vi "test图层-修改中.vi"() -> ()   [LabVIEW 2018]
doc: "This example demonstrates the use of binary morphological reconstruction in the particle analysis. The example allows you to keep the particles completely inside the ROI, completely outside the ROI or on the ROI."
uses:
  <vilib>/vision/NI_Vision_Development_Module.lvlib
panel:
  out "Image Compare":T1(plugin-control)
  out "下":i32
  out "右":i32
  out "上":i32
  out "左":i32
  out "面积":i32
  out "标准差":sgl
  out "平均值":sgl
  out "最大灰度值":sgl
  out "最小灰度值":sgl
  out "选中框灰度表":u32[](graph)
  out "Image Dst Out":T1(plugin-control)
  out "全图灰度级信息":T2 {"标准差" format="%.2f"; "均值" format="%.2f"; "相邻灰度级间隔" format="%.2f"; "起始灰度值" format="%.2f"; "最大值" format="%.2f"; "最小值" format="%.2f"}
  out "图片灰度表":u32[](graph)
  in  "Font, Size & Style 2":T3={"Desired Font (Application)"=enum."Application Font", "[User-specified Font]"={"Font Name"="", "Size"=12, "Strikeout?"=FALSE, "Italic?"=FALSE, "Underline?"=FALSE, "Outline?"=FALSE, "Shadow?"=FALSE, "Bold?"=FALSE, "Rotation Angle"=0.0}, "Horizontal Alignment"=0, "Vertical Alignment"=0} {"Vertical Alignment" items=["Bottom", "Top", "Baseline"]; "Horizontal Alignment" items=["Left", "Center", "Right"]; "[User-specified Font]"."Rotation Angle" format="%.2f"}
  in  "选择框号":bool
  out "当前选择框的编号":dbl
  out "框总数":dbl
  in  "Font, Size & Style":T3={"Desired Font (Application)"=enum."Application Font", "[User-specified Font]"={"Font Name"="", "Size"=12, "Strikeout?"=FALSE, "Italic?"=FALSE, "Underline?"=FALSE, "Outline?"=FALSE, "Shadow?"=FALSE, "Bold?"=FALSE, "Rotation Angle"=0.0}, "Horizontal Alignment"=0, "Vertical Alignment"=0} {"Vertical Alignment" items=["Bottom", "Top", "Baseline"]; "Horizontal Alignment" items=["Left", "Center", "Right"]; "[User-specified Font]"."Rotation Angle" format="%.2f"}
  out "框组":T4(array[cluster])
  in  "单次删除":bool
  in  "Operation":enum16{"overlay rectangle"}(ring)
  out "标注图":T1(plugin-control)
  in  "退出标注":bool
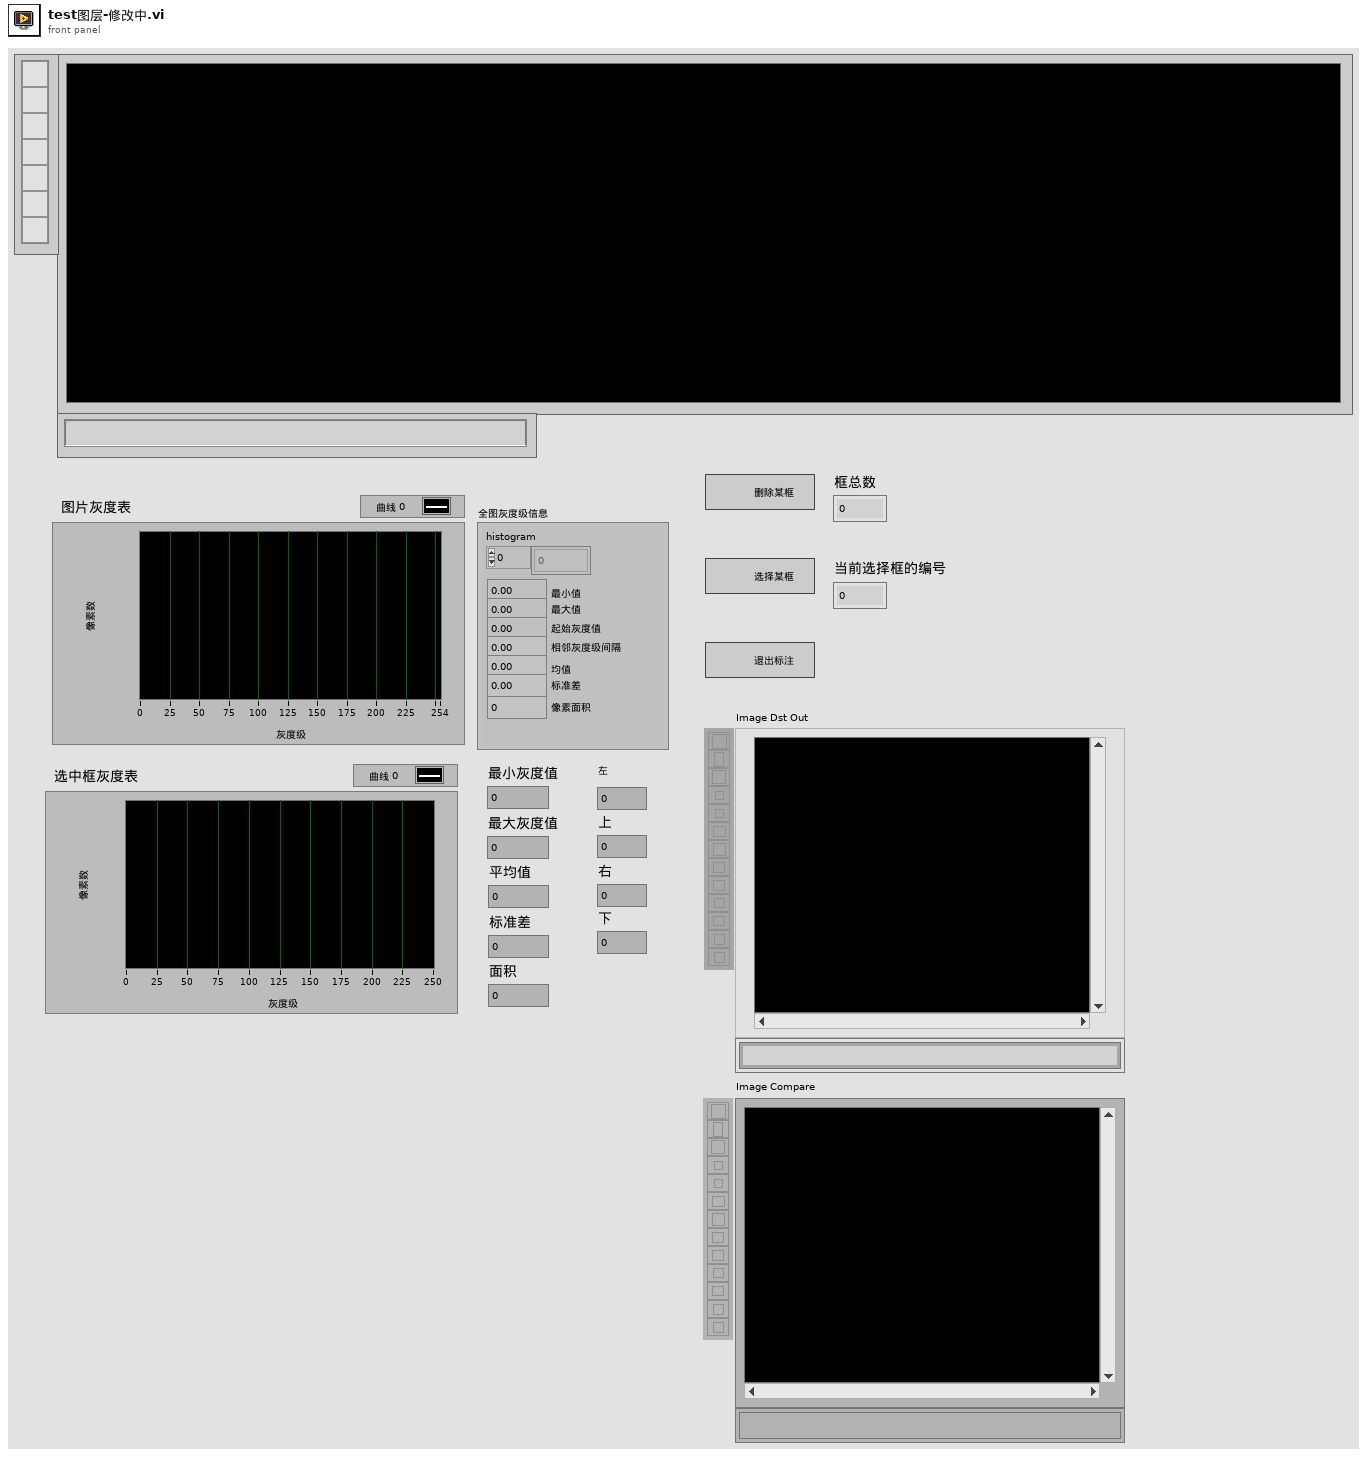
[diagram p1: front panel]
types:
  T1 = typedef "IMAQ Image.ctl" = refnum<image>
  T2 = cluster{"histogram":u32[], "最小值":sgl, "最大值":sgl, "起始灰度值":sgl, "相邻灰度级间隔":sgl, "均值":sgl, "标准差":sgl, "像素面积":i32}
  T3 = cluster{"Desired Font (Application)":enum16{"User-specified Font", "Application Font", "System Font", "Dialog Font"}, "[User-specified Font]":cluster{"Font Name":string, "Size":i16, "Strikeout?":bool, "Italic?":bool, "Underline?":bool, "Outline?":bool, "Shadow?":bool, "Bold?":bool, "Rotation Angle":dbl}, "Horizontal Alignment":i16, "Vertical Alignment":i16}
  T4 = cluster{"Global Rectangle":i32[], "Contours":cluster{"Contour Type":u32, "ROI Type":u32, "Points":i32[]}[]}[]
  T5 = typedef "Image Type" = u32
  T6 = enum32{"Average", "Min", "Max", "Clear  if < ", "Clear  if < or =", "Clear  if =", "Clear  if > or =", "Clear  if >"}
  T7 = cluster{"Global Rectangle":i32[], "Contours":cluster{"Contour Type":u32, "ROI Type":u32, "Points":i32[]}[]}
  T8 = typedef "IMAQ Rectangle" = cluster{"Left":i32, "Top":i32, "Right":i32, "Bottom":i32, "Rotation":dbl}
  T9 = cluster{"histogram":u32[], "Minimal Value":sgl, "Maximal Value":sgl, "Starting Value":sgl, "Interval Width":sgl, "Mean Value":sgl, "Standard  Variation":sgl, "Area (pixels)":i32}
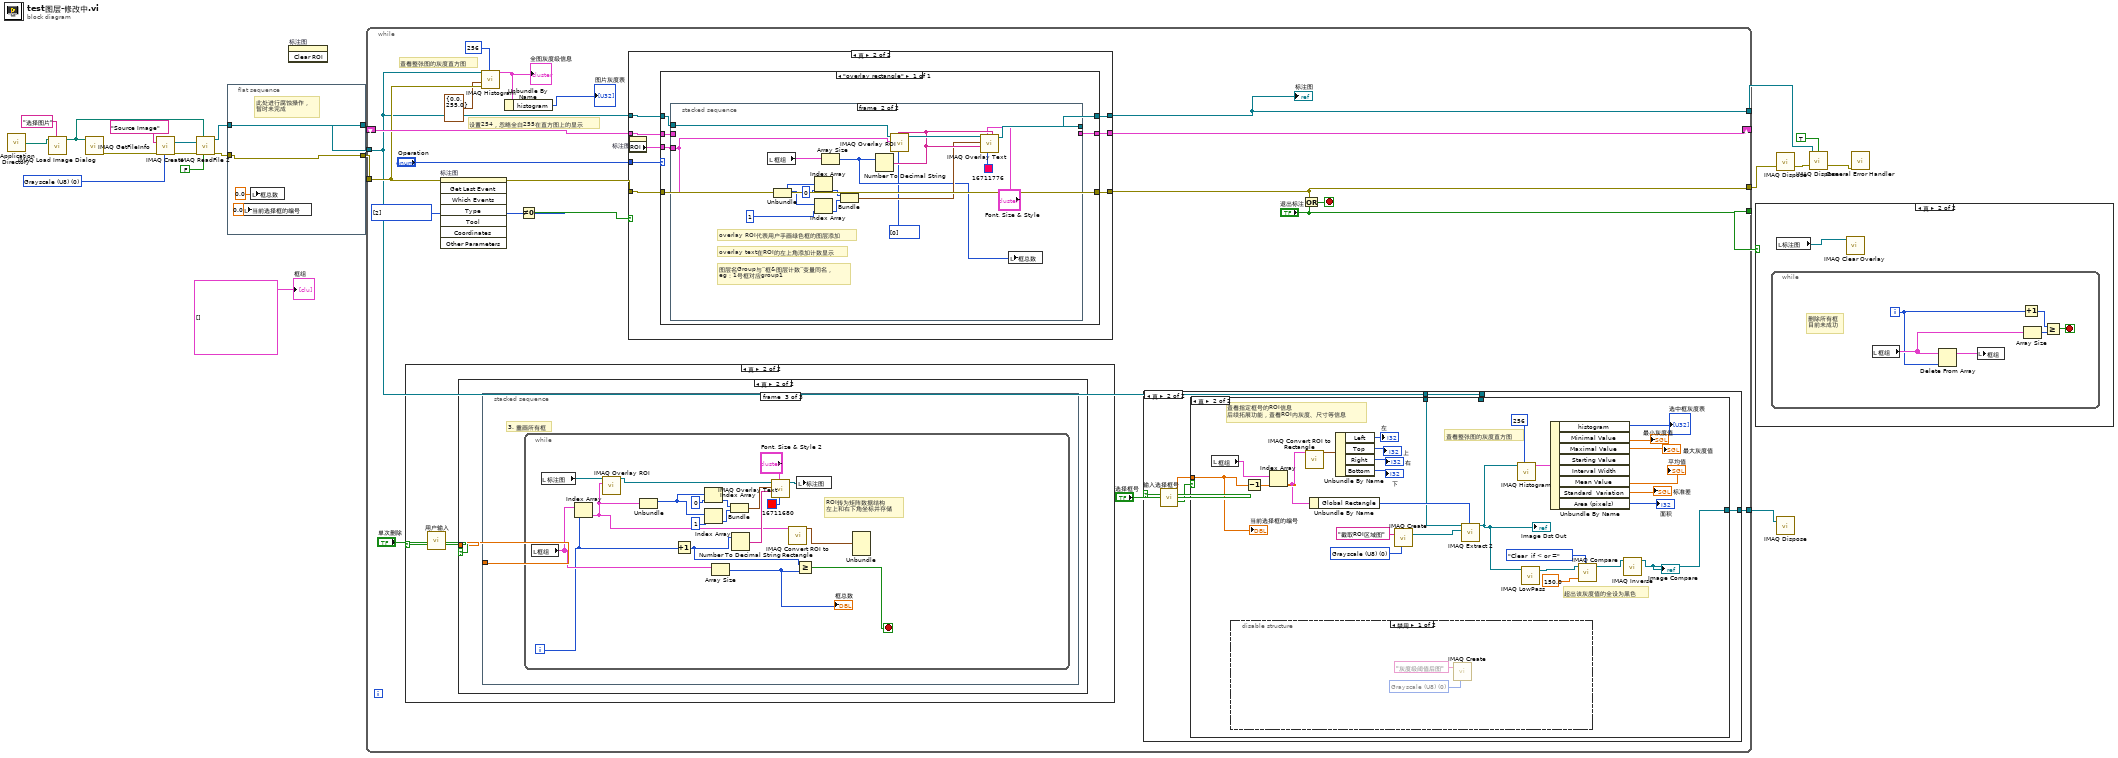
[diagram p0: block diagram]
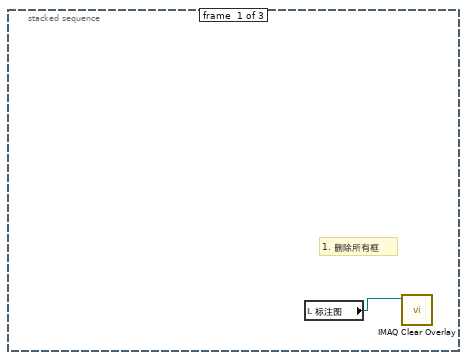
[diagram p8: hidden frame]
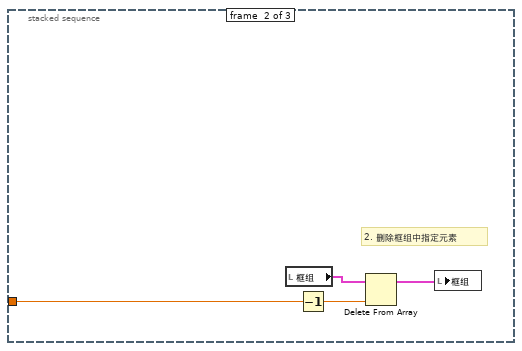
[diagram p9: hidden frame]
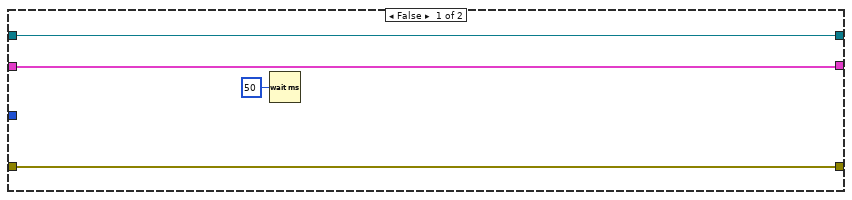
[diagram p10: hidden frame]
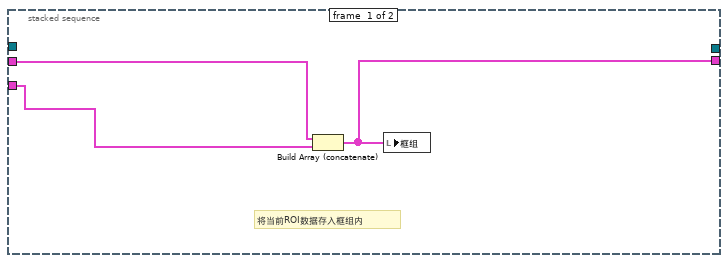
[diagram p11: hidden frame]
diagram:
  w12 = T5 0 items=["Grayscale (U8)", "Grayscale (I16)", "Grayscale (SGL)", "Complex (CSG)", "RGB (U32)", "HSL (U32)", "RGB (U64)", "Grayscale (U16)"] ("Image Type")
  n1 = call <vilib>:"Application Directory.vi"() -> ("Application Directory"=w13:path)
  n2 = call "IMAQ Load Image Dialog"("Prompt"="选择图片" ("prompt"), "Start Path"=w13) -> ("Path"=w19:path)  [unwired: 7 in, 2 out]
  n3 = call "IMAQ GetFileInfo"("File Path"=w19) -> ("error out"=w17:errorcluster)  [unwired: 4 in, 6 out]
  n4 = call "IMAQ Create"("Image Name"="Source Image", "Image Type"=w12, "error in (no error)"=w17) -> ("New Image"=w15:T1, "error out"=w14:errorcluster)  [unwired: 2 in]
  n5 = call "IMAQ ReadFile 2"("Use File Path Image Type"=FALSE, "File Path"=w19, "error in (no error)"=w14, "Image"=w15) -> ("error out"=w4:errorcluster, "Image Out"=w2:T1)  [unwired: 3 in, 3 out]
  n6 = flat-sequence {
    tunnel: [w23] -> w3
    tunnel: w4 -> [w23]
    tunnel: w2 -> [w22]
    tunnel: [w22] -> w1
    frame #0 {
      # "此处进行腐蚀操作，\n暂时未完成"
      n7 = local write "当前选择框的编号"(0.0 ("当前框的编号")) -> ()
      n8 = local write "框总数"(0.0 ("框总数")) -> ()
    }
  }
  n9 = invoke on="标注图" class="ImageControl" method="Clear ROI"() -> ()  [unwired: 3 in, 3 out]
  n10 = while {
    tunnel: [w28] -> w10
    tunnel: [w41] -> w8
    shift-right: [w37] -> _
    shift-left: _ -> [w36]
    tunnel: ["退出标注"] -> w20
    tunnel: w3 -> [w33]
    tunnel: [w27] -> w5
    tunnel: w1 -> [w26]
    stop <- w40 stop-if-true
    w43 = i32[] [2] items=["No Event"=0, "Click Event"=1, "Draw Event"=2, "Size Event"=4, "Scroll Event"=5, "Double Click Event"=8] ("Which Events")
    # "设置254，忽略全白255在直方图上的显示"
    # "查看整张图的灰度直方图"
    n11 = case shown="真" "单次删除" {
      frame False {
      }
      frame True {
        n12 = call "用户输入"() -> ("框号"=w83:dbl, "确定"=w84:bool)  [unwired: 17 in, 1 out]
        n13 = case shown="真" w84 {
          tunnel: w83 -> [_ w85]
          frame False {
            # "用户取消操作"
          }
          frame True {
            n14 = stacked-sequence {
              tunnel: w85 -> [_ w89 _]
              frame #0 {
                # "1. 删除所有框"
                n15 = local read "标注图"() -> (w86:T1)
                n16 = call "IMAQ Clear Overlay"("Image"=w86) -> ()  [unwired: 9 in, 2 out]
              }
              frame #1 {
                # "2. 删除框组中指定元素"
                n17 = local read "框组"() -> (w90:T4)
                n18 = Decrement(x=w89) -> (x-1=w88:dbl)
                n19 = Delete From Array(array=w90, index=w88) -> (array with subset deleted=w87:T4)  [unwired: 1 in, 1 out]
                n20 = local write "框组"(w87) -> ()
              }
              frame #2 {
                # "3. 重画所有框"
                n21 = while {
                  i -> [w94]
                  stop <- w109 stop-if-true
                  # "ROI转为矩阵数据结构\n左上和右下角坐标并存储"
                  n22 = local read "框组"() -> (w102:T4)
                  n23 = local read "标注图"() -> (w108:T1)
                  n24 = Index Array(array=w102, index=w94) -> (element=w95:T7)
                  n25 = call "IMAQ Overlay ROI"("ROI Descriptor"=w95, "Image"=w108) -> ("Image Out"=w104:T1)  [unwired: 8 in, 1 out]
                  n26 = Unbundle(w95) -> ("Global Rectangle"=w98:i32[])  [unwired: 1 out]
                  n27 = Increment(x=w94) -> (x+1=w107:i32)
                  n28 = Index Array(array=w98, index=0 ("索引")) -> (element=w99:i32)
                  n29 = Index Array(array=w98, index=1 ("索引")) -> (element=w100:i32)
                  n30 = Array Size(array=w102) -> (size(s)=w92:i32)
                  "框总数" <- w92
                  n31 = Bundle(w99, w100) -> (w97:cluster{i32, i32})  [unwired: 1 in]
                  n32 = Number To Decimal String(number=w107) -> (decimal integer string=w105:string)  [unwired: 1 in]
                  n33 = call "IMAQ Overlay Text"("Text Color (black)"=u32 16711680, "Font, Size & Style"="Font, Size & Style 2", "String"=w105, "Origin"=w97, "Image"=w104) -> ("Image Out"=w103:T1)  [unwired: 5 in, 1 out]
                  n34 = call "IMAQ Convert ROI to Rectangle"("ROI Descriptor"=w95) -> ("Rectangle"=w93:T8)  [unwired: 8 in, 1 out]
                  n35 = Greater Or Equal?(x=w107, y=w92) -> (x >= y?=w109:bool)
                  n36 = local write "标注图"(w103) -> ()
                  n37 = Unbundle(w93) -> ()  [unwired: 5 out]
                }
              }
            }
          }
        }
      }
    }
    n38 = invoke on="标注图" class="ImageControl" method="Get Last Event"(error in=w33, "Which Events"=w43) -> (error out=w42:errorcluster, "Type"=w44:i32)  [unwired: 6 in, 6 out]
    n39 = call "IMAQ Histogram"("Number of Classes"=256, "error in (no error)"=w33, "Interval Range"=cluster{"Minimum":sgl, "Maximum":sgl} {"Minimum"=0.0, "Maximum"=255.0}, "Image"=w26) -> ("Histogram Report"=w30:T9)  [unwired: 6 in, 1 out]
    "全图灰度级信息" <- w30
    n40 = Unbundle By Name(w30) -> ("histogram"=→"图片灰度表":u32[])
    n41 = Not Equal To 0?(x=w44) -> (x != 0?=w38:bool)
    n42 = case shown="真" w38 {
      tunnel: w26 -> [w113 w121]
      tunnel: [w113 w120] -> w28
      tunnel: "Operation" -> [_ w118]
      tunnel: w42 -> [w112 w117]
      tunnel: [w112 w116] -> w41
      tunnel: [w110 w115] -> w37
      tunnel: w36 -> [w110 w114]
      frame False {
        n43 = Wait (ms)(milliseconds to wait=u32 50) -> ()  [unwired: 1 out]
      }
      frame True {
        n44 = property on="标注图" class="ImageControl"() -> ("ROI"=w119:T7)  [unwired: 2 in, 2 out]
        n45 = case shown="\"overlay rectangle\"" w118 {
          tunnel: w121 -> [w126]
          tunnel: w119 -> [w124]
          tunnel: [w125] -> w120
          tunnel: w117 -> [w127]
          tunnel: [w127] -> w116
          tunnel: [w123] -> w115
          tunnel: w114 -> [w122]
          frame "overlay rectangle" {
            n46 = stacked-sequence {
              tunnel: w126 -> [_ w137]
              tunnel: [_ w136] -> w125
              tunnel: w124 -> [w130 w133]
              tunnel: [w128 _] -> w123
              tunnel: w122 -> [w129 _]
              frame #0 {
                # "将当前ROI数据存入框组内"
                n47 = Build Array (concatenate)(w129, w130) -> (w128:T4)
                n48 = local write "框组"(w128) -> ()
              }
              frame #1 {
                # "图层名Group与“框&图层计数”变量同名，\neg：1号框对应group1"
                # "overlay text在ROI的左上角添加计数显示"
                # "overlay ROI代表用户手画绿色框的图层添加"
                n49 = local read "框组"() -> (w142:T4)
                n50 = Unbundle(w133) -> ("Global Rectangle"=w145:i32[])  [unwired: 1 out]
                n51 = Index Array(array=w145, index=0 ("索引")) -> (element=w144:i32)
                n52 = Index Array(array=w145, index=1 ("索引")) -> (element=w143:i32)
                n53 = Array Size(array=w142) -> (size(s)=w132:i32)
                n54 = Bundle(w144, w143) -> (w135:cluster{i32, i32})  [unwired: 1 in]
                n55 = Number To Decimal String(number=w132) -> (decimal integer string=w141:string)  [unwired: 1 in]
                n56 = call "IMAQ Overlay ROI"("Colors (Green)"=u32[] [0], "Group"=w141, "ROI Descriptor"=w133, "Image"=w137) -> ("Image Out"=w146:T1)  [unwired: 6 in, 1 out]
                n57 = call "IMAQ Overlay Text"("Group"=w141, "Text Color (black)"=u32 16711776, "Font, Size & Style"="Font, Size & Style", "String"=w141, "Origin"=w135, "Image"=w146) -> ("Image Out"=w136:T1)  [unwired: 4 in, 1 out]
                n58 = local write "框总数"(w132) -> ()
              }
            }
          }
        }
      }
    }
    "标注图" <- w28
    n59 = case shown="真" "选择框号" {
      tunnel: [w46 w49] -> w27
      tunnel: w26 -> [_ w48]
      tunnel: w26 -> [w46 w47]
      frame False {
      }
      frame True {
        n60 = call "输入选择框号"() -> ("框号"=w50:dbl, "确定"=w51:bool)  [unwired: 17 in, 1 out]
        n61 = case shown="真" w51 {
          tunnel: w50 -> [_ w79]
          tunnel: [w52 w53] -> w49
          tunnel: w48 -> [_ w60]
          tunnel: w47 -> [w52 _]
          frame False {
            # "用户取消操作"
          }
          frame True {
            w76 = T5 0 items=["Grayscale (U8)", "Grayscale (I16)", "Grayscale (SGL)", "Complex (CSG)", "RGB (U32)", "HSL (U32)", "RGB (U64)", "Grayscale (U16)"] ("Image Type")
            # "超出该灰度值的全设为黑色"
            # "查看整张图的灰度直方图"
            # "查看指定框号的ROI信息\n后续拓展功能，查看ROI内灰度、尺寸等信息"
            n62 = local read "框组"() -> (w78:T4)
            n63 = disable-structure shown="禁用" {
              frame Disabled {
                w81 = T5 0 items=["Grayscale (U8)", "Grayscale (I16)", "Grayscale (SGL)", "Complex (CSG)", "RGB (U32)", "HSL (U32)", "RGB (U64)", "Grayscale (U16)"] ("Image Type")
                n64 = call "IMAQ Create"("Image Name"="灰度级阈值后图", "Image Type"=w81) -> ()  [unwired: 3 in, 2 out]
              }
              frame Enabled {
              }
            }
            n65 = Decrement(x=w79) -> (x-1=w80:dbl)
            n66 = Index Array(array=w78, index=w80) -> (element=w59:T7)
            n67 = call "IMAQ Convert ROI to Rectangle"("ROI Descriptor"=w59) -> ("Rectangle"=w65:T8)  [unwired: 8 in, 1 out]
            n68 = Unbundle By Name(w59) -> ("Global Rectangle"=w77:i32[])
            n69 = Unbundle By Name(w65) -> ("Left"=→"左":i32, "Top"=→"上":i32, "Right"=→"右":i32, "Bottom"=→"下":i32)
            n70 = call "IMAQ Create"("Image Name"="截取ROI区域图", "Image Type"=w76) -> ("New Image"=w74:T1)  [unwired: 3 in, 1 out]
            n71 = call "IMAQ Extract 2"("Optional Rectangle"=w77, "Image Dst"=w74, "Image Src"=w60) -> ("Image Dst Out"=w56:T1)  [unwired: 7 in, 1 out]
            "Image Dst Out" <- w56
            n72 = call "IMAQ Histogram"("Number of Classes"=256, "Image"=w56) -> ("Histogram Report"=w72:T9)  [unwired: 8 in, 1 out]
            n73 = call "IMAQ LowPass"("Image Src"=w56) -> ("Image Dst Out"=w57:T1)  [unwired: 6 in, 1 out]
            n74 = Unbundle By Name(w72) -> ("histogram"=→"选中框灰度表":u32[], "Minimal Value"=→"最小灰度值":sgl, "Maximal Value"=→"最大灰度值":sgl, "Mean Value"=→"平均值":sgl, "Standard  Variation"=→"标准差":sgl, "Area (pixels)"=→"面积":i32)  [unwired: 2 out]
            n75 = call "IMAQ Compare"("Constant"=sgl 150.0 ("筛选灰度阈值下限"), "Operator"=T6."Clear  if < or =", "Image Src A"=w57) -> ("Image Dst Out"=w54:T1)  [unwired: 7 in, 1 out]
            n76 = call "IMAQ Inverse"("Image Src"=w54) -> ("Image Dst Out"=w53:T1)  [unwired: 9 in, 1 out]
            "Image Compare" <- w53
            "当前选择框的编号" <- w79
          }
        }
      }
    }
    n77 = Or(x=w41, y="退出标注") -> (x .or. y?=w40:bool)
  }
  n78 = case shown="真" w20 {
    frame False {
    }
    frame True {
      n79 = while {
        i -> [w152]
        stop <- w149 stop-if-true
        # "删除所有框\n目前未成功"
        n80 = local read "框组"() -> (w153:T4)
        n81 = Delete From Array(array=w153, index=w152) -> (array with subset deleted=w148:T4)  [unwired: 1 in, 1 out]
        n82 = local write "框组"(w148) -> ()
        n83 = Increment(x=w152) -> (x+1=w151:i32)
        n84 = Array Size(array=w153) -> (size(s)=w150:i32)
        n85 = Greater Or Equal?(x=w151, y=w150) -> (x >= y?=w149:bool)
      }
      n86 = local read "标注图"() -> (w147:T1)
      n87 = call "IMAQ Clear Overlay"("Image"=w147) -> ()  [unwired: 9 in, 2 out]
    }
  }
  n88 = call "IMAQ Dispose"("error in (no error)"=w8) -> ("error out"=w9:errorcluster)  [unwired: 2 in, 3 out]
  n89 = call "IMAQ Dispose"("Image"=w5) -> ()  [unwired: 2 in, 4 out]
  n90 = call "IMAQ Dispose"("All Images? (No)"=TRUE, "Image"=w10, "error in (no error)"=w9) -> ("error out"=w7:errorcluster)  [unwired: 3 out]
  n91 = call <vilib>:"General Error Handler.vi"("error in (no error)"=w7) -> ()  [unwired: 10 in, 5 out]
  "框组" <- T4 [] ("框组")
